vi "Combine secondary hit coinc results.vi"(11 "secondary hits array":T2(array[cluster])) -> (3 "Combined secondaries":T1(array[cluster]))   [LabVIEW 2016]
uses:
  Global Variables/System info.vi
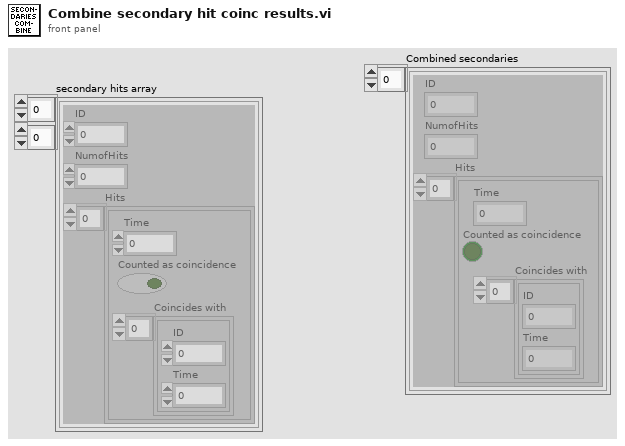
[diagram p1: front panel]
types:
  T1 = cluster{"ID":i8, "NumofHits":i32, "Hits":cluster{"Time":u64, "Counted as coincidence":bool, "Coincides with":cluster{"ID":i8, "Time":u64}[]}[]}[]
  T2 = cluster{"ID":i8, "NumofHits":i32, "Hits":cluster{"Time":u64, "Counted as coincidence":bool, "Coincides with":cluster{"ID":i8, "Time":u64}[]}[]}[][]
  T3 = cluster{"ID":i8, "NumofHits":i32, "Hits":cluster{"Time":u64, "Counted as coincidence":bool, "Coincides with":cluster{"ID":i8, "Time":u64}[]}[]}
  T4 = cluster{"Time":u64, "Counted as coincidence":bool, "Coincides with":cluster{"ID":i8, "Time":u64}[]}
  T5 = cluster{"Time":u64, "Counted as coincidence":bool, "Coincides with":cluster{"ID":i8, "Time":u64}[]}[]
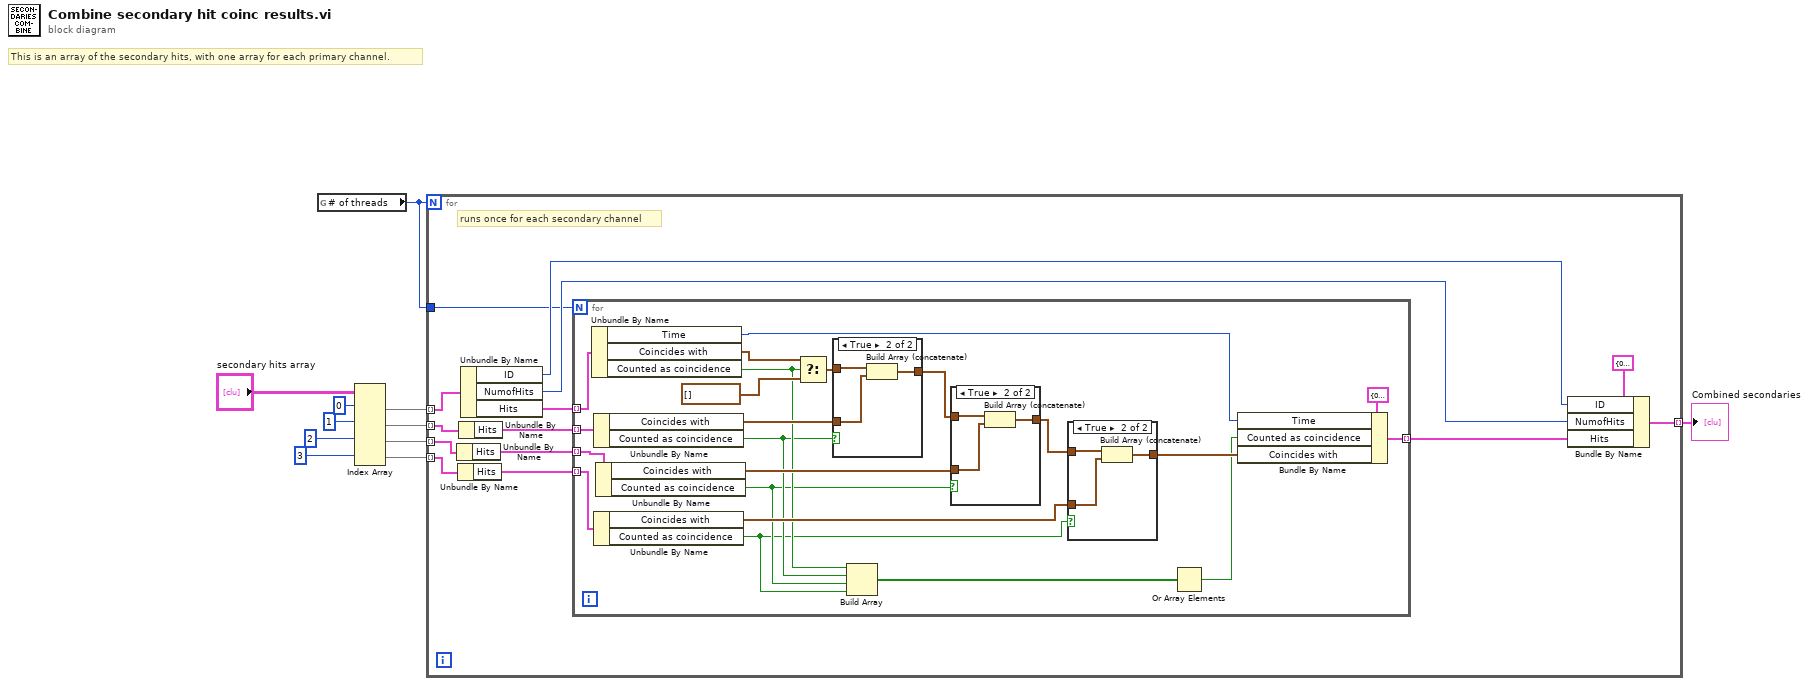
[diagram p0: block diagram]
diagram:
  # "This is an array of the secondary hits, with one array for each primary channel."
  n1 = global read "System info.vi" "# of threads"() -> (w2:i32)
  n2 = Index Array(array="secondary hits array", index (row) #1=0 ("index (row)"), index (row) #2=1 ("index (row)"), index (row) #3=2 ("index (row)"), index (row) #4=3 ("index (row)")) -> (element #1=w6:T1, element #2=w5:T1, element #3=w4:T1, element #4=w3:T1)  [unwired: 4 in]
  n3 = for {
    N: w2 -> [_]
    tunnel: w6 -> [w25] mode=indexing
    tunnel: w5 -> [w24] mode=indexing
    tunnel: w4 -> [w22] mode=indexing
    tunnel: w3 -> [w23] mode=indexing
    tunnel: [w13] -> w1 mode=indexing
    tunnel: w2 -> [w12]
    # "runs once for each secondary channel"
    n4 = Unbundle By Name(w22) -> ("Hits"=w19:T5)
    n5 = Unbundle By Name(w23) -> ("Hits"=w18:T5)
    n6 = Unbundle By Name(w24) -> ("Hits"=w20:T5)
    n7 = Unbundle By Name(w25) -> ("ID"=w14:i8, "NumofHits"=w15:i32, "Hits"=w21:T5)
    n8 = for {
      N: w12 -> [_]
      tunnel: w21 -> [w47] mode=indexing
      tunnel: w20 -> [w44] mode=indexing
      tunnel: w19 -> [w41] mode=indexing
      tunnel: w18 -> [w37] mode=indexing
      tunnel: [w26] -> w16 mode=indexing
      n9 = Unbundle By Name(w47) -> ("Time"=w34:u64, "Coincides with"=w46:cluster{"ID":i8, "Time":u64}[], "Counted as coincidence"=w32:bool)
      n10 = Unbundle By Name(w44) -> ("Coincides with"=w42:cluster{"ID":i8, "Time":u64}[], "Counted as coincidence"=w31:bool)
      n11 = Unbundle By Name(w37) -> ("Coincides with"=w36:cluster{"ID":i8, "Time":u64}[], "Counted as coincidence"=w29:bool)
      n12 = Unbundle By Name(w41) -> ("Coincides with"=w40:cluster{"ID":i8, "Time":u64}[], "Counted as coincidence"=w30:bool)
      n13 = Select(t=w46, s=w32, f=cluster{"ID":i8, "Time":u64}[] []) -> (s? t:f=w43:cluster{"ID":i8, "Time":u64}[])
      n14 = case shown="True" w31 {
        tunnel: w43 -> [w56 w59]
        tunnel: w42 -> [_ w58]
        tunnel: [w56 w57] -> w39
        frame False {
        }
        frame True {
          n15 = Build Array (concatenate)(w59, w58) -> (w57:cluster{"ID":i8, "Time":u64}[])
        }
      }
      n16 = Build Array(w32, w31, w30, w29) -> (w28:bool[])
      n17 = case shown="True" w30 {
        tunnel: w39 -> [w52 w55]
        tunnel: w40 -> [_ w54]
        tunnel: [w52 w53] -> w38
        frame False {
        }
        frame True {
          n18 = Build Array (concatenate)(w55, w54) -> (w53:cluster{"ID":i8, "Time":u64}[])
        }
      }
      n19 = case shown="True" w29 {
        tunnel: w38 -> [w48 w51]
        tunnel: w36 -> [_ w50]
        tunnel: [w48 w49] -> w33
        frame False {
        }
        frame True {
          n20 = Build Array (concatenate)(w51, w50) -> (w49:cluster{"ID":i8, "Time":u64}[])
        }
      }
      n21 = Or Array Elements(Boolean array=w28) -> (logical OR=w27:bool)
      n22 = Bundle By Name(cluster=T4 {"Time"=0, "Counted as coincidence"=FALSE, "Coincides with"=[]}, "Time"=w34, "Counted as coincidence"=w27, "Coincides with"=w33) -> (w26:T4)
    }
    n23 = Bundle By Name(cluster=T3 {"ID"=0, "NumofHits"=0, "Hits"=[]} ("Cluster"), "ID"=w14, "NumofHits"=w15, "Hits"=w16) -> (w13:T3)
  }
  "Combined secondaries" <- w1
